vi "R(T) T(t) SETP(t) with ramp332 DC ramp current(File overwrite Fixed)_1.vi"(0 "I":dbl=1e-06 min=1e-09 max=1.0 step=1e-06 format="%.4e", 1 "Ti":dbl min=0.0 max=400.0 format="%.3f", 2 "Tf":dbl=4.0 min=0.0 max=400.0 format="%.3f", 3 "Ramp":ext format="%.3f", 4 "Range":dbl=3.0 format="%.2f", 7 "Measurement":bool=TRUE, 8 "Auto\nTemp?":bool=TRUE) -> ()   [LabVIEW 2013]
uses:
  subVIs/Control 1.ctl
panel:
  in  "Y data precision":T1=7.0
  in  "X data precision":T1=3.0
  in  "Path":path
  in  "File name":string
  out "T(t)":cluster{"X":dbl, "Y":dbl}[](graph)
  in  "Autorange":bool=TRUE
  in  "Volt Delay":u32=50
  in  "Voltmeter PLC":dbl=1.0 min=0.01 max=60.0 step=0.01 format="%.2f"
  in  "Voltage Compliance":dbl=12.0 min=0.1 max=105.0 step=0.1 format="%.2f"
  in  "minutes to wait before start":u32=5
  out "R/Ohm":dbl=1e-09 min=-1.0 step=1e-09 format="%.3e"
  out "T/K":dbl min=0.0 step=0.01 format="%.3f"
  out "?":cluster{dbl, dbl}[](graph)
  in  "Delay time":sgl min=0 step=1 format="%.2f"
  # "ON"
  # "OFF"
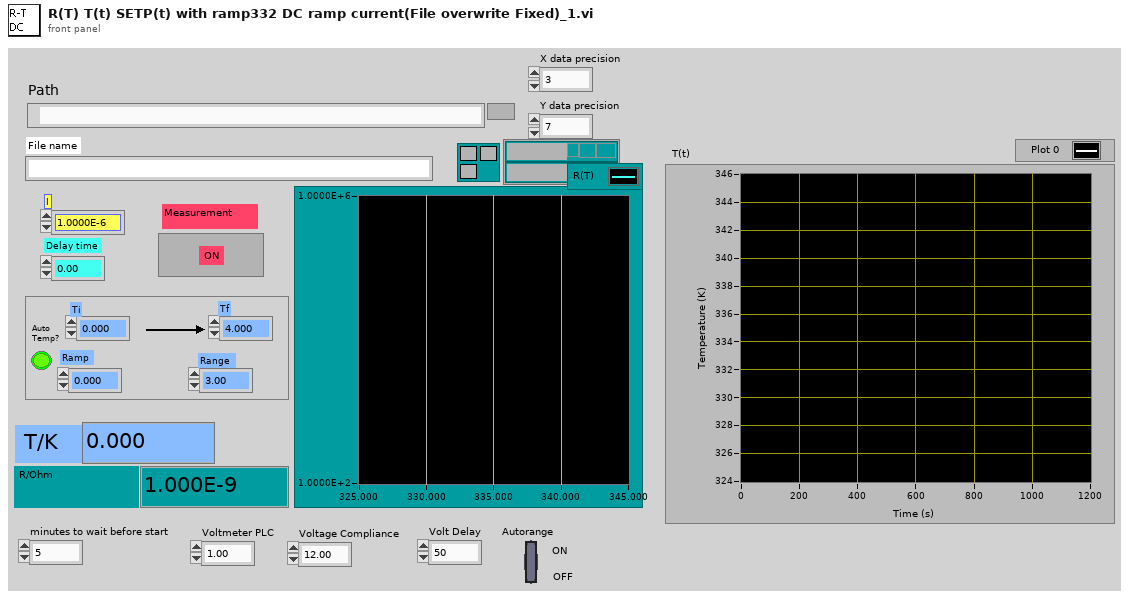
[diagram p1: front panel]
types:
  T1 = typedef "Control 1.ctl" = dbl
  T2 = enum16{"open", "replace", "create", "open or create", "replace or create", "replace or create with confirmation"}
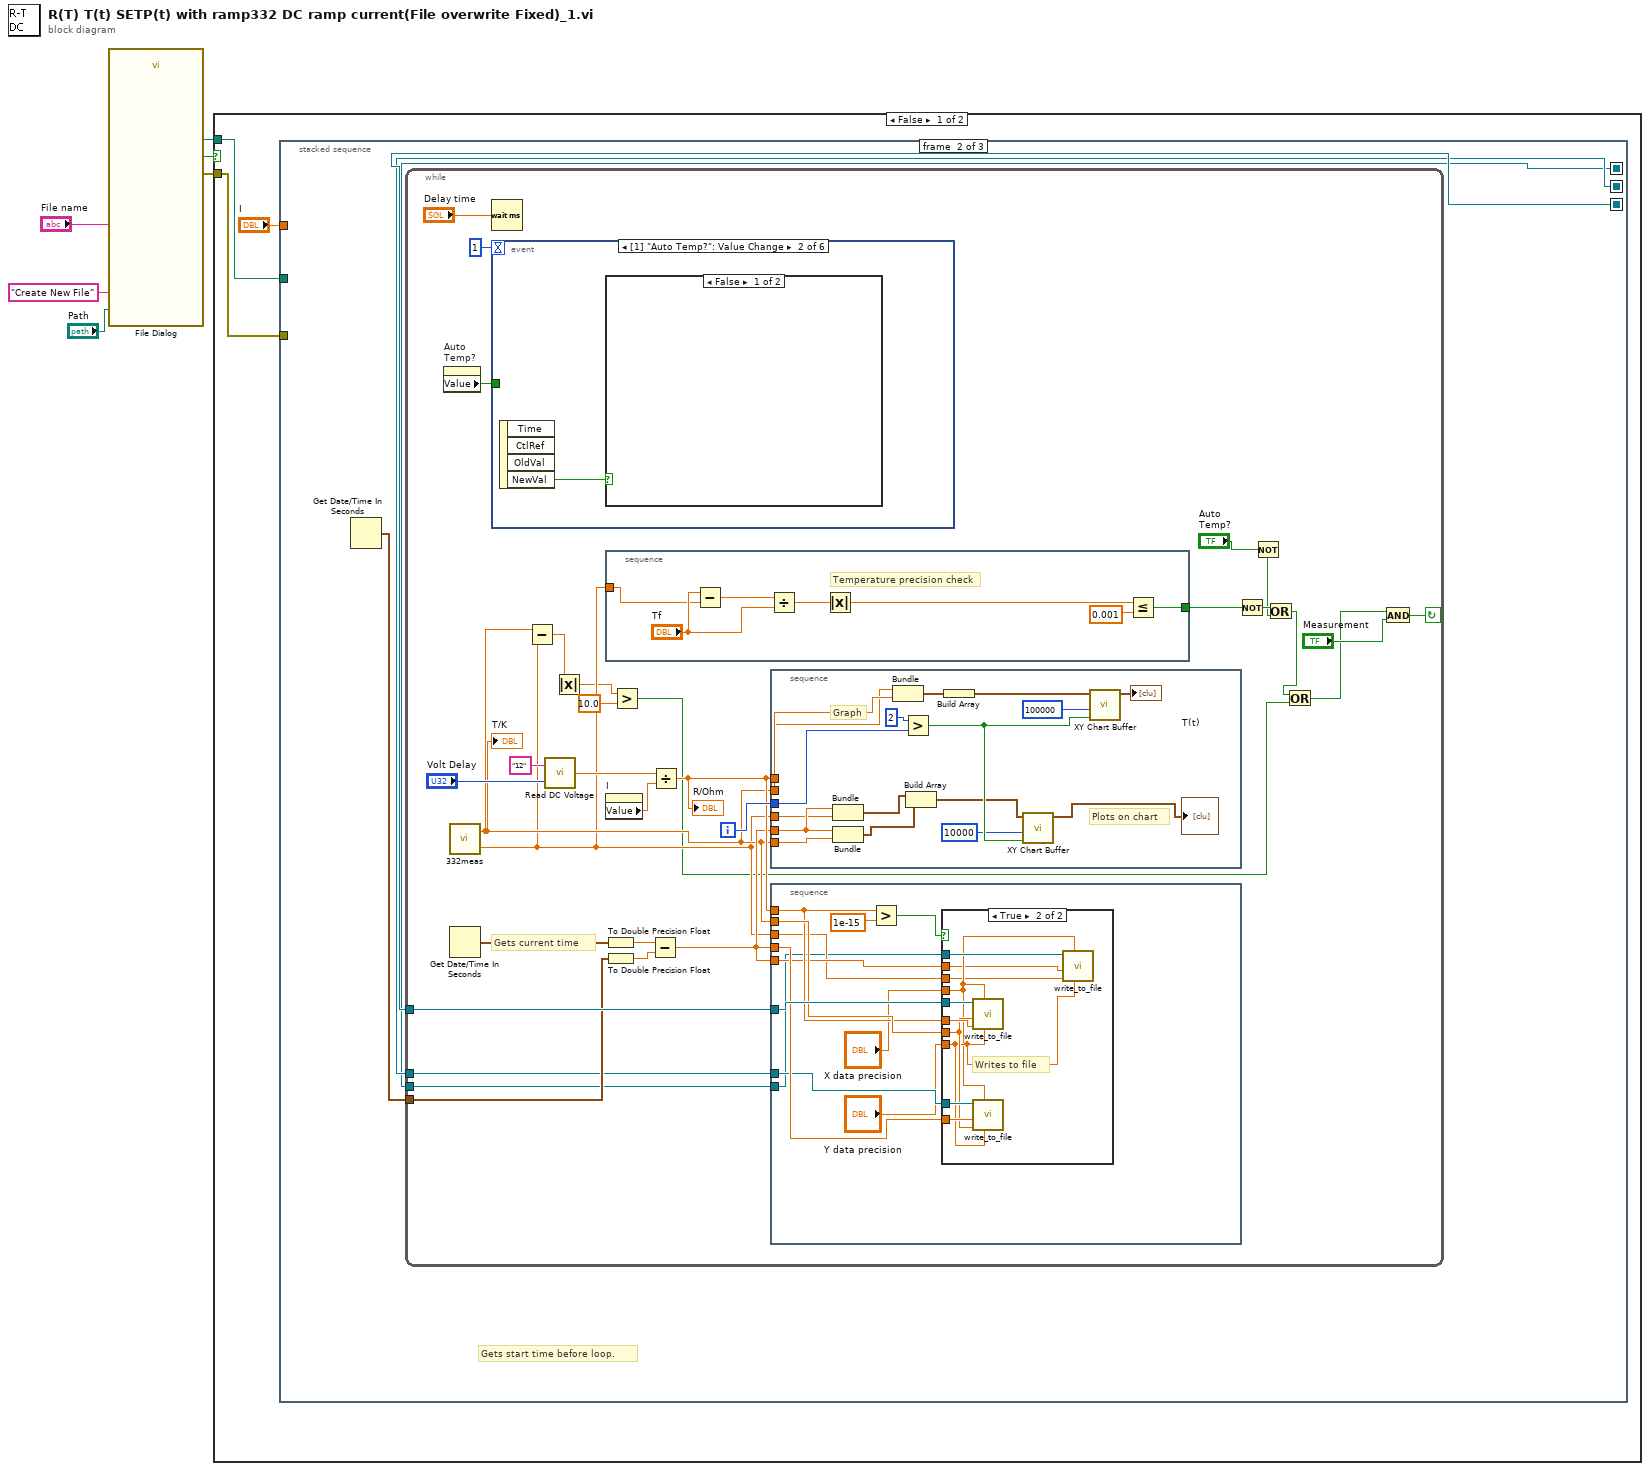
[diagram p0: block diagram]
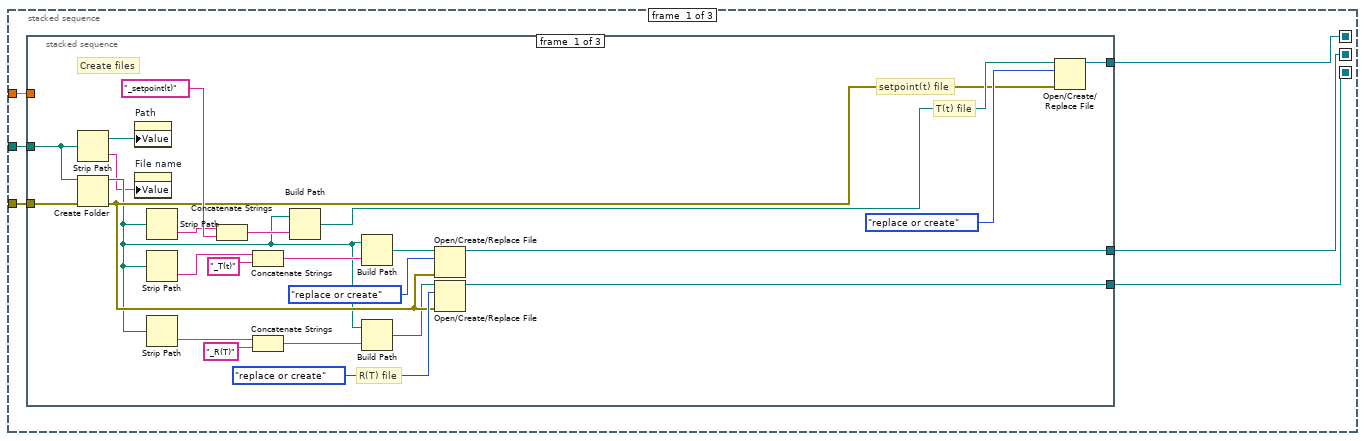
[diagram p2: hidden frame]
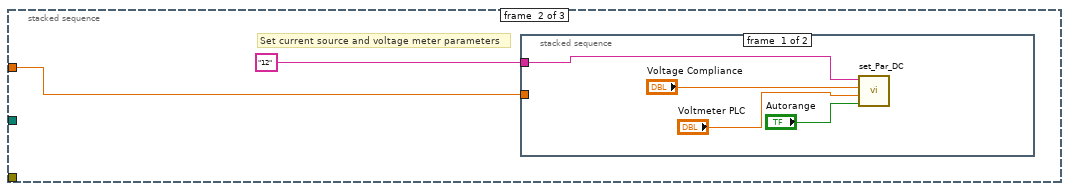
[diagram p3: hidden frame]
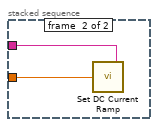
[diagram p4: hidden frame]
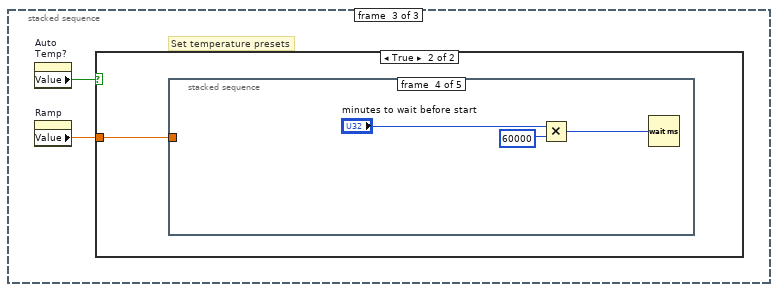
[diagram p5: hidden frame]
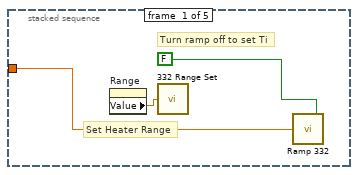
[diagram p7: hidden frame]
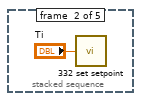
[diagram p8: hidden frame]
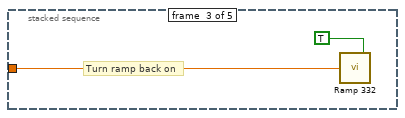
[diagram p9: hidden frame]
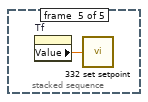
[diagram p10: hidden frame]
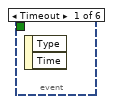
[diagram p12: hidden frame]
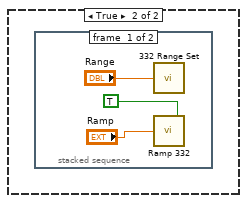
[diagram p13: hidden frame]
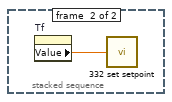
[diagram p14: hidden frame]
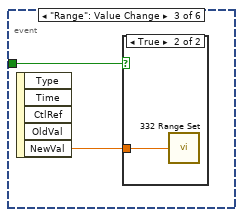
[diagram p15: hidden frame]
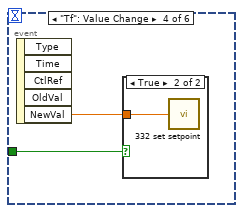
[diagram p17: hidden frame]
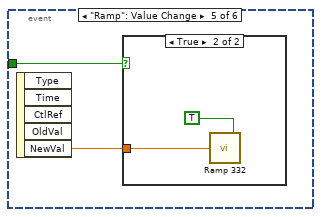
[diagram p19: hidden frame]
diagram:
  n1 = call "File Dialog"("start path"="Path", "prompt"="Create New File", "default name"="File name") -> ("selected path"=w3:path, "cancelled"=w1:bool, "error out"=w2:errorcluster)  [unwired: 9 in, 1 out]
  n2 = case shown="False" w1 {
    tunnel: w3 -> [w9 _]
    tunnel: w2 -> [w8 _]
    frame False {
      n3 = stacked-sequence {
        seq-local: [w15 _ _] -> [_ w64 w165]
        seq-local: [w13 _ _] -> [_ w62 w161]
        seq-local: [w12 _ _] -> [_ w61 _]
        tunnel: "I" -> [w14 _ w162]
        tunnel: w9 -> [w11 _ _]
        tunnel: w8 -> [w10 _ _]
        frame #0 {
          n4 = stacked-sequence {
            tunnel: [w39 _ _] -> w15
            tunnel: w14 -> [_ w40 _]
            tunnel: [w36 _ _] -> w13
            tunnel: [w26 _ _] -> w12
            tunnel: w11 -> [w19 _ _]
            tunnel: w10 -> [w18 _ _]
            frame #0 {
              # "setpoint(t) file"
              # "T(t) file"
              # "R(T) file"
              # "Create files"
              n5 = Strip Path(path=w19) -> (stripped path=w16:path, name=w17:string)
              n6 = Create Folder(path (use dialog)=w19, error in=w18) -> (created path=w23:path, error out=w25:errorcluster)  [unwired: 1 in, 1 out]
              n7 = property on="Path" class="Path"("Value"=w16) -> ()  [unwired: 2 in, 2 out]
              n8 = property on="File name" class="Str"("Value"=w17) -> ()  [unwired: 2 in, 2 out]
              n9 = Strip Path(path=w23) -> (name=w28:string)  [unwired: 1 out]
              n10 = Strip Path(path=w23) -> (name=w35:string)  [unwired: 1 out]
              n11 = Strip Path(path=w23) -> (name=w21:string)  [unwired: 1 out]
              n12 = Concatenate Strings(w28, "_setpoint(t)" ("name or relative path")) -> (w30:string)
              n13 = Concatenate Strings(w35, "_T(t)" ("name or relative path")) -> (w33:string)
              n14 = Concatenate Strings(w21, "_R(T)" ("name or relative path")) -> (w20:string)
              n15 = Build Path(base path=w23, name or relative path=w30) -> (appended path=w31:path)
              n16 = Build Path(base path=w23, name or relative path=w33) -> (appended path=w32:path)
              n17 = Build Path(base path=w23, name or relative path=w20) -> (appended path=w24:path)
              n18 = Open/Create/Replace File(file path (use dialog)=w32, error in=w25, operation (0:open)=T2."replace or create") -> (refnum out=w36:refnum<file>)  [unwired: 3 in, 2 out]
              n19 = Open/Create/Replace File(file path (use dialog)=w24, error in=w25, operation (0:open)=T2."replace or create") -> (refnum out=w39:refnum<file>)  [unwired: 3 in, 2 out]
              n20 = Open/Create/Replace File(file path (use dialog)=w31, error in=w25, operation (0:open)=T2."replace or create") -> (refnum out=w26:refnum<file>)  [unwired: 3 in, 2 out]
            }
            frame #1 {
              # "Set current source and voltage meter parameters"
              n21 = stacked-sequence {
                tunnel: "12" ("Address") -> [w45 w47]
                tunnel: w40 -> [_ w46]
                frame #0 {
                  n22 = call "set_Par_DC.vi"("Autorange"="Autorange", "Voltmeter PLC"="Voltmeter PLC", "Voltage Compliance"="Voltage Compliance", "Address"=w45) -> ()
                }
                frame #1 {
                  n23 = call "Set DC Current Ramp.vi"("Address"=w47, "Current"=w46) -> ()
                }
              }
            }
            frame #2 {
              # "Set temperature presets"
              n24 = property on="Auto\nTemp?" class="Bool (strict)"() -> ("Value"=w49:bool)  [unwired: 2 in, 2 out]
              n25 = property on="Ramp" class="DigNum (strict)"() -> ("Value"=w48:ext)  [unwired: 2 in, 2 out]
              n26 = case shown="True" w49 {
                tunnel: w48 -> [_ w50]
                frame False {
                }
                frame True {
                  n27 = stacked-sequence {
                    tunnel: w50 -> [w52 _ w56 _ _]
                    frame #0 {
                      # "Set Heater Range"
                      # "Turn ramp off to set Ti"
                      n28 = property on="Range" class="DigNum (strict)"() -> ("Value"=w51:dbl)  [unwired: 2 in, 2 out]
                      n29 = call "332 Range Set.vi"("Power Range: 93C\n0=OFF, 1=Low, 2=Med, 3=High"=w51) -> ()
                      n30 = call "Ramp 332.vi"("On"=FALSE, "K/min"=w52) -> ()
                    }
                    frame #1 {
                      n31 = call "332 set setpoint.vi"("Set Temperature SetPoint:332"="Ti") -> ()
                    }
                    frame #2 {
                      # "Turn ramp back on"
                      n32 = call "Ramp 332.vi"("On"=TRUE, "K/min"=w56) -> ()
                    }
                    frame #3 {
                      n33 = Multiply(x="minutes to wait before start", y=u32 60000) -> (x*y=w58:u32)
                      n34 = Wait (ms)(milliseconds to wait=w58) -> ()  [unwired: 1 out]
                    }
                    frame #4 {
                      n35 = property on="Tf" class="DigNum (strict)"() -> ("Value"=w60:dbl)  [unwired: 2 in, 2 out]
                      n36 = call "332 set setpoint.vi"("Set Temperature SetPoint:332"=w60) -> ()
                    }
                  }
                }
              }
            }
          }
        }
        frame #1 {
          # "Gets start time before loop."
          n37 = Get Date/Time In Seconds() -> (seconds since 1Jan1904=w63:timestamp)
          n38 = while {
            tunnel: w64 -> [w92]
            tunnel: w63 -> [w76]
            tunnel: w62 -> [w75]
            tunnel: w61 -> [w73]
            i -> [w95]
            stop <- w94 continue-if-true
            # "Gets current time"
            n39 = property on="Auto\nTemp?" class="Bool (strict)"() -> ("Value"=w89:bool)  [unwired: 2 in, 2 out]
            n40 = call "332meas.vi"() -> ("332 Temp [K]"=w72:dbl, "332 Temp Setpoint [K]"=w71:dbl)  [unwired: 1 in]
            "T/K" <- w72
            n41 = Get Date/Time In Seconds() -> (seconds since 1Jan1904=w78:timestamp)
            n42 = Wait (ms)(milliseconds to wait="Delay time") -> ()  [unwired: 1 out]
            n43 = event shown="[1] \"Auto Temp?\": Value Change" {
              selector: _ -> [_ _ _ _ _ _]
              dyn-events: _ -> [_ _ _ _ _ _]
              timeout: 1 -> [_ _ _ _ _ _]
              tunnel: w89 -> [_ _ w148 w150 w153 _]
              event Timeout {
                n44 = event-data() -> ()  [unwired: 1 in, 2 out]
              }
              event "Auto\nTemp?": Value Change {
                n45 = event-data() -> ("NewVal"=w142:bool)  [unwired: 1 in, 3 out]
                n46 = case shown="False" w142 {
                  frame False {
                  }
                  frame True {
                    n47 = stacked-sequence {
                      frame #0 {
                        n48 = call "332 Range Set.vi"("Power Range: 93C\n0=OFF, 1=Low, 2=Med, 3=High"="Range") -> ()
                        n49 = call "Ramp 332.vi"("On"=TRUE, "K/min"="Ramp") -> ()
                      }
                      frame #1 {
                        n50 = property on="Tf" class="DigNum (strict)"() -> ("Value"=w146:dbl)  [unwired: 2 in, 2 out]
                        n51 = call "332 set setpoint.vi"("Set Temperature SetPoint:332"=w146) -> ()
                      }
                    }
                  }
                }
              }
              event "Range": Value Change {
                n52 = event-data() -> ("NewVal"=w147:dbl)  [unwired: 1 in, 4 out]
                n53 = case shown="True" w148 {
                  tunnel: w147 -> [_ w149]
                  frame False {
                  }
                  frame True {
                    n54 = call "332 Range Set.vi"("Power Range: 93C\n0=OFF, 1=Low, 2=Med, 3=High"=w149) -> ()
                  }
                }
              }
              event "Tf": Value Change {
                n55 = event-data() -> ("NewVal"=w151:dbl)  [unwired: 1 in, 4 out]
                n56 = case shown="True" w150 {
                  tunnel: w151 -> [_ w152]
                  frame False {
                  }
                  frame True {
                    n57 = call "332 set setpoint.vi"("Set Temperature SetPoint:332"=w152) -> ()
                  }
                }
              }
              event "Ramp": Value Change {
                n58 = event-data() -> ("NewVal"=w154:ext)  [unwired: 1 in, 4 out]
                n59 = case shown="True" w153 {
                  tunnel: w154 -> [_ w155]
                  frame False {
                  }
                  frame True {
                    n60 = call "Ramp 332.vi"("On"=TRUE, "K/min"=w155) -> ()
                  }
                }
              }
              event "I": Value Change {
                n61 = event-data() -> ("NewVal"=w157:dbl)  [unwired: 1 in, 4 out]
                n62 = stacked-sequence {
                  tunnel: w157 -> [_ w159]
                  frame #0 {
                    # "Wait until measurement\nfinished"
                    n63 = Wait (ms)(milliseconds to wait=u32 1000) -> ()  [unwired: 1 out]
                  }
                  frame #1 {
                    n64 = call "Set DC Current.vi"("Address"="24" ("address string"), "Current"=w159) -> ()
                  }
                }
              }
            }
            n65 = Subtract(x=w72, y=w71) -> (x-y=w70:dbl)
            n66 = call "Read DC Voltage.vi"("Volt Delay"="Volt Delay", "Address"="12" ("address string")) -> ("Voltage"=w81:dbl)
            n67 = Absolute Value(x=w70) -> (abs(x)=w66:dbl)
            n68 = stacked-sequence {
              tunnel: [w136] -> w93
              tunnel: w71 -> [w135]
              frame #0 {
                # "Temperature precision check"
                n69 = Subtract(x="Tf", y=w135) -> (x-y=w139:dbl)
                n70 = Divide(x=w139, y="Tf") -> (x/y=w140:dbl)
                n71 = Absolute Value(x=w140) -> (abs(x)=w138:dbl)
                n72 = Less Or Equal?(x=w138, y=0.001) -> (x <= y?=w136:bool)
              }
            }
            n73 = property on="I" class="DigNum (strict)"() -> ("Value"=w82:dbl)  [unwired: 2 in, 2 out]
            n74 = To Double Precision Float(number=w78) -> (double precision float=w79:dbl)
            n75 = To Double Precision Float(number=w76) -> (double precision float=w77:dbl)
            n76 = Greater?(x=w66, y=10.0) -> (0:w65:bool)
            n77 = Subtract(x=w79, y=w77) -> (x-y=w74:dbl)
            n78 = Divide(x=w81, y=w82) -> (x/y=w84:dbl)
            "R/Ohm" <- w84
            n79 = stacked-sequence {
              tunnel: w95 -> [w108]
              tunnel: w84 -> [w106]
              tunnel: w72 -> [w105]
              tunnel: w74 -> [w103]
              tunnel: w72 -> [w104]
              tunnel: w71 -> [w102]
              frame #0 {
                # "Plots on chart"
                # "Graph"
                n80 = Bundle(w103, "332 Temp Setpoint [K]"=w102) -> (w101:cluster{dbl, "332 Temp Setpoint [K]":dbl})  [unwired: 1 in]
                n81 = Bundle(w103, "332 Temp [K]"=w104) -> (w96:cluster{dbl, "332 Temp [K]":dbl})  [unwired: 1 in]
                n82 = Bundle("332 Temp [K]"=w105, w106) -> (w112:cluster{"332 Temp [K]":dbl, dbl})  [unwired: 1 in]
                n83 = Greater?(x=2, y=w108) -> (0:w100:bool)
                n84 = Build Array(w101, w96) -> (w98:cluster{dbl, "332 Temp [K]":dbl}[])
                n85 = Build Array(w112) -> (w110:cluster{"332 Temp [K]":dbl, dbl}[])
                n86 = call "XY Chart Buffer.vi"("clear first (no:F)"=w100, "chart length (points)"=10000, "new points"=w98) -> ("XY chart data"=→"T(t)":cluster{"x":dbl, "y":dbl}[])  [unwired: 8 in]
                n87 = call "XY Chart Buffer.vi"("clear first (no:F)"=w100, "chart length (points)"=100000, "new points"=w110) -> ("XY chart data"=→"?":cluster{"x":dbl, "y":dbl}[])  [unwired: 8 in]
              }
            }
            n88 = stacked-sequence {
              tunnel: w92 -> [w124]
              tunnel: w84 -> [w122]
              tunnel: w72 -> [w123]
              tunnel: w74 -> [w119]
              tunnel: w75 -> [w118]
              tunnel: w74 -> [w117]
              tunnel: w71 -> [w116]
              tunnel: w73 -> [w115]
              frame #0 {
                n89 = Greater?(x=w122, y=1e-15) -> (0:w121:bool)
                n90 = case shown="True" w121 {
                  tunnel: w124 -> [_ w133]
                  tunnel: w122 -> [_ w132]
                  tunnel: w123 -> [_ w129]
                  tunnel: w119 -> [_ w130]
                  tunnel: w118 -> [_ w131]
                  tunnel: w117 -> [_ w125]
                  tunnel: w116 -> [_ w126]
                  tunnel: w115 -> [_ w134]
                  tunnel: "Y data precision" -> [_ w128]
                  tunnel: "X data precision" -> [_ w127]
                  frame False {
                  }
                  frame True {
                    # "Writes to file"
                    n91 = call "write_to_file.vi"("y data precision"=w128, "x data precision"=w127, "y data"=w132, "x data"=w129, "refnum"=w133) -> ()  [unwired: 6 in]
                    n92 = call "write_to_file.vi"("y data precision"=w128, "x data precision"=w127, "y data"=w129, "x data"=w130, "refnum"=w131) -> ()  [unwired: 6 in]
                    n93 = call "write_to_file.vi"("y data precision"=w128, "x data precision"=w127, "y data"=w126, "x data"=w125, "refnum"=w134) -> ()  [unwired: 6 in]
                  }
                }
              }
            }
            n94 = Not(x=w93) -> (.not. x?=w90:bool)
            n95 = Not(x="Auto\nTemp?") -> (.not. x?=w85:bool)
            n96 = Or(x=w90, y=w85) -> (x .or. y?=w69:bool)
            n97 = Or(x=w69, y=w65) -> (x .or. y?=w68:bool)
            n98 = And(x=w68, y="Measurement") -> (x .and. y?=w94:bool)
          }
        }
        frame #2 {
          w163 = "12" ("Address")
          n99 = stacked-sequence {
            tunnel: w163 -> [w167 w168]
            tunnel: w162 -> [w166 _]
            frame #0 {
              n100 = call "Set DC Current Ramp to Zero.vi"("Address"=w167, "Current"=w166) -> ()
            }
            frame #1 {
              n101 = call "disarm.vi"("address string"=w168) -> ()  [unwired: 1 in, 1 out]
            }
          }
          n102 = call "Send to Volt Meter.vi"("Address"=w163, "Data"=":trig:sour imm;:init") -> ()
          n103 = Close File(refnum=w161) -> ()  [unwired: 1 in, 2 out]
          n104 = Close File(refnum=w165) -> ()  [unwired: 1 in, 2 out]
        }
      }
    }
    frame True {
    }
  }
